vi "To Serial Form.vi"(6 "Serial Version":T1, 10 "Serializer in":refnum<class "Serializer.lvclass">, 11 "Test in":refnum<class "Test.lvclass">) -> (0 "error out":errorcluster, 2 "Serializer out":refnum<class "Serializer.lvclass">, 3 "Test out":refnum<class "Test.lvclass">)   [LabVIEW 2014, in "Test.lvclass"]
uses:
  Test.lvclass
  <vilib>/NI/AQ Character Lineator/Serializable/Serializable.lvclass
  <vilib>/NI/AQ Character Lineator/Serializable/Insert Data Value Reference of Serializable.vi
  <vilib>/NI/AQ Character Lineator/Serializer/Serializer.lvclass
  <vilib>/NI/AQ Character Lineator/Serialization Common/Serial Version.ctl
  <vilib>/NI/AQ Character Lineator/Serialization Common/Serialization Common.lvlib
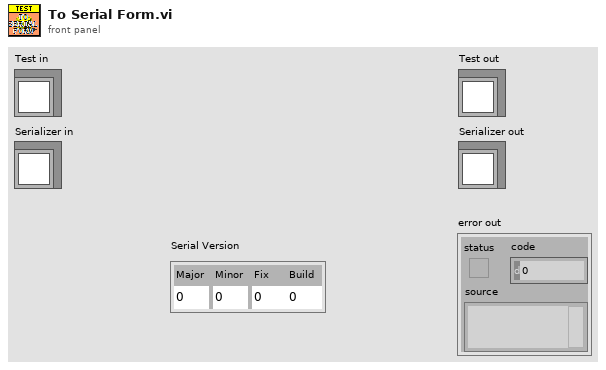
[diagram p1: front panel]
types:
  T1 = typedef "Serialization Common.lvlib/Serial Version.ctl" = cluster{"Major":u16, "Minor":u16, "Fix":u16, "Build":u16}
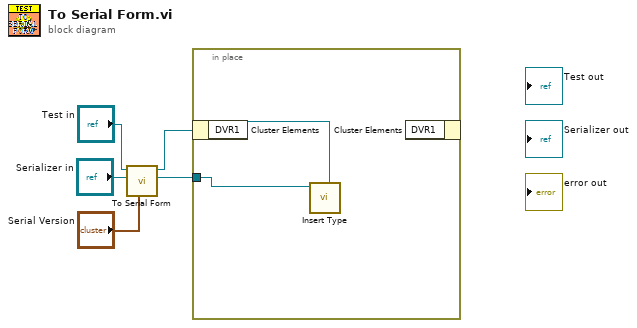
[diagram p0: block diagram]
diagram:
  n1 = call-parent "To Serial Form.vi"("Serial Version"="Serial Version", "Serializer in"="Serializer in", "Serializable in"="Test in") -> ("Serializer out"=w2:refnum<class "Serializer.lvclass">, "Serializable out"=w1:refnum<class "Test.lvclass">)  [unwired: 6 in, 1 out]
  n2 = in-place {
    in-place-border: w2 -> [w7]
    n3 = in-place-cluster #1(w1) -> ("DVR1"=w6:refnum<data-value>)
    n4 = call-poly <vilib>:"Insert Type.vi"("Reference"=w6, "Serializer in"=w7) -> ()  [unwired: 8 in, 2 out]
    n5 = in-place-cluster #1() -> ()  [unwired: 1 in, 1 out]
  }
